vi "6300 laser sweep and oscilloscope.vi"() -> ()   [LabVIEW 2011]
uses:
  <vilib>/Instr/_visa.llb/VISA Open Access Mode.ctl
panel:
  in  "Oscilloscope wait time (ms)":u32
  in  "laser wait time (ms)":u32=1100
  in  "Oscilloscope read time (ms)":u32=4000
  out "error out 2":errorcluster
  in  "Oscilloscope VISA GPIB Resource":refnum<visa-resource-name>="GPIB0::7::INSTR"
  out "error out":errorcluster
  out "WavelengthMin":dbl=1519.01 format="%.2f"
  out "WavelengthMax":dbl=1570.29 format="%.2f"
  out "MaxSlewRate":dbl=23.9 format="%.2f"
  in  "StartSweep":bool
  in  "ReturnSlewrate":dbl=23.9 format="%.2f"
  in  "ForwardSlewrate":dbl=23.9 format="%.2f"
  in  "StopWavelength":dbl=1570.29 format="%.2f"
  in  "StartWavelength":dbl=1519.01 format="%.2f"
  in  "resource name (\"\")":string="GPIB0::10::INSTR"
  # "Sweep Example\n\nStart program with above arrow.\nSet parameters and press StartSweep.\nLaser will reset to the start wavelength then sweep to the stop wavelength."
  # "Min"
  # "Max"
  # "Max"
  # "Set up for GPIB address 1.  Change as needed."
  # "Reference Value:\nFor 2.2s, 4Msa/s:\nlaser wait time: 1100ms;\noscilloscope read time: 4000ms;\n\nFor 2s, 400Ksa/s;\nlaser wait time: 1000ms \noscilloscope read time: \n\nFor 5s, 5Mpts oscilloscope setting:\nlaser wait time: 2600ms;\nOscilloscope read time: 8000ms;\n\nFor 20s, 10Mpts setting:\nlaser wait time: 10500ms;\nOscilloscope read time: 35000ms;\nf\nFor 50s, 200Ksa/s setting:\nlaser wait time: 25000ms\nOscilloscope read time: 85000ms;\nChannel offset:\nCH1:\nCH2:\nCH3:\nCH4:"
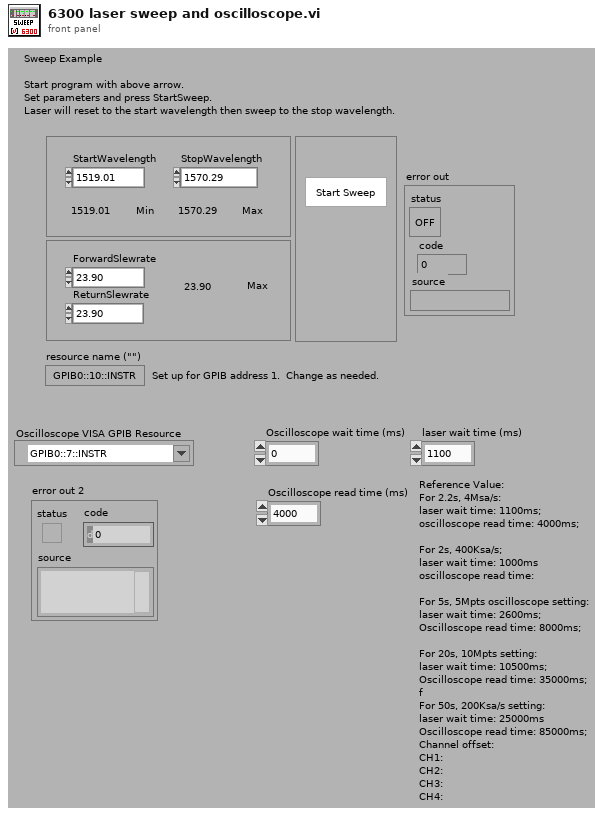
[diagram p1: front panel]
types:
  T1 = enum16{"Diode Current", "Diode Temperature", "Piezo Volt", "Wavelength", "Forward Slew Rate", "Return Slew Rate", "Scan Start Wavelength", "Scan Stop Wavelength", "MaxSlewRate", "Wavelength Max", "Wavelength Min"}
  T2 = enum16{"Diode Current", "Diode Temperature", "Piezo Volt", "Wavelength", "Forward Slewrate", "Return Slewrate", "Scan Start Wavelength", "Scan Stop Wavelength", "Wavelength Max", "Wavelength Min", "Constant Power On", "Constant Power Off"}
  T3 = enum16{"Scan Reset", "Scan Start", "Scan Stop", "Laser On", "Laser Off", "Laser State?", "Track Off"}
  T4 = enum16{"Identification Query", "Operation Complete Query"}
  T5 = typedef "VISA Open Access Mode.ctl" = u32
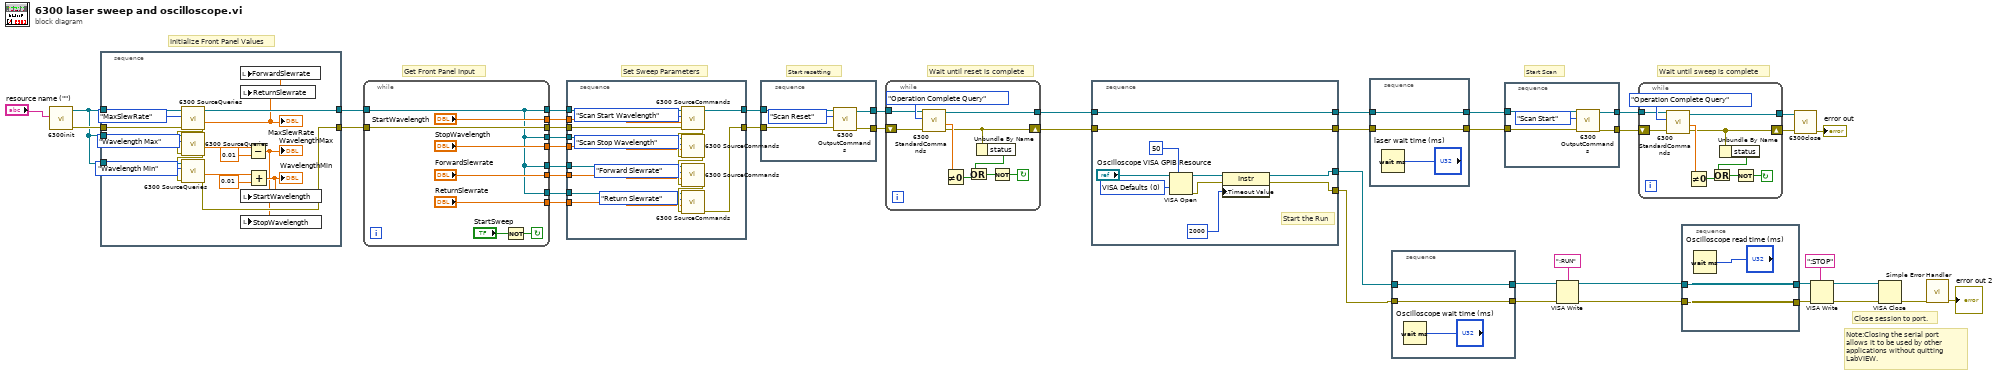
[diagram p0: block diagram]
diagram:
  # "Note:Closing the serial port allows it to be used by other applications without quitting LabVIEW."
  # "Close session to port."
  # "Initialize Front Panel Values"
  # "Wait until sweep is complete"
  # "Start Scan"
  # "Wait until reset is complete"
  # "Start resetting"
  # "Set Sweep Parameters"
  # "Get Front Panel Input"
  n1 = call <instrlib>:"6300init.vi"("resource name (\"\")"="resource name (\"\")") -> ("error out"=w25:errorcluster, "dup VISA session"=w22:refnum<visa-resource-name>)  [unwired: 9 in]
  n2 = stacked-sequence {
    tunnel: w22 -> [w57]
    tunnel: w25 -> [w56]
    tunnel: [w57] -> w24
    tunnel: [w51] -> w23
    tunnel: w22 -> [w55]
    tunnel: w22 -> [w54]
    frame #0 {
      n3 = call <instrlib>:"6300 SourceQueries.VI"("error in"=w56, "Setpoint to Query?"=T1."MaxSlewRate", "VISA session"=w57) -> ("error out"=w53:errorcluster, "Returned Number"=w44:dbl)  [unwired: 5 in, 2 out]
      "MaxSlewRate" <- w44
      n4 = call <instrlib>:"6300 SourceQueries.VI"("error in"=w53, "Setpoint to Query?"=T1."Wavelength Max", "VISA session"=w55) -> ("error out"=w52:errorcluster, "Returned Number"=w47:dbl)  [unwired: 5 in, 2 out]
      n5 = call <instrlib>:"6300 SourceQueries.VI"("error in"=w52, "Setpoint to Query?"=T1."Wavelength Min", "VISA session"=w54) -> ("error out"=w51:errorcluster, "Returned Number"=w48:dbl)  [unwired: 5 in, 2 out]
      n6 = local write "ForwardSlewrate"(w44) -> ()
      n7 = local write "ReturnSlewrate"(w44) -> ()
      n8 = Subtract(x=w47, y=0.01) -> (x-y=w45:dbl)
      "WavelengthMax" <- w45
      n9 = local write "StopWavelength"(w45) -> ()
      n10 = Add(x=w48, y=0.01) -> (x+y=w46:dbl)
      "WavelengthMin" <- w46
      n11 = local write "StartWavelength"(w46) -> ()
    }
  }
  n12 = while {
    tunnel: [w61] -> w34
    tunnel: [w61] -> w35
    tunnel: [w61] -> w36
    tunnel: [w61] -> w37
    tunnel: ["ReturnSlewrate"] -> w39
    tunnel: ["ForwardSlewrate"] -> w40
    tunnel: ["StopWavelength"] -> w41
    tunnel: ["StartWavelength"] -> w42
    tunnel: [w68] -> w38
    tunnel: w23 -> [w68]
    tunnel: w24 -> [w61]
    stop <- w62 continue-if-true
    n13 = Not(x="StartSweep") -> (.not. x?=w62:bool)
  }
  n14 = stacked-sequence {
    tunnel: w42 -> [w83]
    tunnel: w41 -> [w82]
    tunnel: w40 -> [w81]
    tunnel: w39 -> [w80]
    tunnel: w38 -> [w79]
    tunnel: [w78] -> w32
    tunnel: w37 -> [w77]
    tunnel: w36 -> [w76]
    tunnel: w35 -> [w75]
    tunnel: w34 -> [w74]
    tunnel: [w73] -> w33
    frame #0 {
      n15 = call <instrlib>:"6300 SourceCommands.VI"("error in"=w79, "Num Com Parameter"=w83, "Source Command?"=T2."Scan Start Wavelength", "VISA session"=w77) -> ("error out"=w86:errorcluster, "dup VISA session"=w73:refnum<visa-resource-name>)  [unwired: 4 in, 2 out]
      n16 = call <instrlib>:"6300 SourceCommands.VI"("error in"=w86, "Num Com Parameter"=w82, "Source Command?"=T2."Scan Stop Wavelength", "VISA session"=w76) -> ("error out"=w85:errorcluster)  [unwired: 4 in, 3 out]
      n17 = call <instrlib>:"6300 SourceCommands.VI"("error in"=w85, "Num Com Parameter"=w81, "Source Command?"=T2."Forward Slewrate", "VISA session"=w75) -> ("error out"=w84:errorcluster)  [unwired: 4 in, 3 out]
      n18 = call <instrlib>:"6300 SourceCommands.VI"("error in"=w84, "Num Com Parameter"=w80, "Source Command?"=T2."Return Slewrate", "VISA session"=w74) -> ("error out"=w78:errorcluster)  [unwired: 4 in, 3 out]
    }
  }
  n19 = stacked-sequence {
    tunnel: w33 -> [w91]
    tunnel: w32 -> [w90]
    tunnel: [w88] -> w31
    tunnel: [w87] -> w30
    frame #0 {
      n20 = call <instrlib>:"6300 OutputCommands.VI"("error in"=w90, "Output Command?"=T3."Scan Reset", "VISA session"=w91) -> ("error out"=w88:errorcluster, "dup VISA session"=w87:refnum<visa-resource-name>)  [unwired: 3 in, 4 out]
    }
  }
  n21 = while {
    tunnel: [w94] -> w13
    tunnel: w30 -> [w98]
    shift-left: w31 -> [w97]
    shift-right: [w93] -> w12
    stop <- w96 continue-if-true
    n22 = call <instrlib>:"6300 StandardCommands.VI"("error in"=w97, "System Command?"=T4."Operation Complete Query", "VISA session"=w98) -> ("error out"=w93:errorcluster, "Returned Number"=w99:dbl, "dup VISA session"=w94:refnum<visa-resource-name>)  [unwired: 5 in, 1 out]
    n23 = Not Equal To 0?(x=w99) -> (x != 0?=w100:bool)
    n24 = Unbundle By Name(w93) -> ("status"=w92:bool)
    n25 = Or(x=w92, y=w100) -> (x .or. y?=w95:bool)
    n26 = Not(x=w95) -> (.not. x?=w96:bool)
  }
  n27 = stacked-sequence {
    tunnel: w13 -> [w111]
    tunnel: [w111] -> w11
    tunnel: w12 -> [w110]
    tunnel: [w110] -> w9
    tunnel: [w103] -> w7
    tunnel: [w102] -> w6
    frame #0 {
      w109 = T5 0 items=["VISA Defaults"=0, "Exclusive Lock"=1, "Load Configured Settings"=4] ("Access Mode")
      # "Start the Run"
      n28 = VISA Open(timeout (0)=u32 50 ("VISA Open timeout (0)"), access mode=w109, VISA resource name="Oscilloscope VISA GPIB Resource") -> (VISA resource name=w106:refnum<visa-resource-name>, error out=w107:errorcluster)  [unwired: 2 in]
      n29 = property class="Instr"(reference=w106, error in=w107, "General Settings:Timeout Value"=u32 2000) -> (reference out=w103:refnum<visa-resource-name>, error out=w102:errorcluster)
    }
  }
  n30 = stacked-sequence {
    tunnel: w11 -> [w113]
    tunnel: [w113] -> w10
    tunnel: w9 -> [w112]
    tunnel: [w112] -> w8
    frame #0 {
      n31 = Wait (ms)(milliseconds to wait="laser wait time (ms)") -> ()  [unwired: 1 out]
    }
  }
  n32 = stacked-sequence {
    tunnel: w7 -> [w116]
    tunnel: [w116] -> w3
    tunnel: w6 -> [w115]
    tunnel: [w115] -> w4
    frame #0 {
      n33 = Wait (ms)(milliseconds to wait="Oscilloscope wait time (ms)") -> ()  [unwired: 1 out]
    }
  }
  n34 = stacked-sequence {
    tunnel: w10 -> [w122]
    tunnel: w8 -> [w121]
    tunnel: [w119] -> w28
    tunnel: [w118] -> w29
    frame #0 {
      n35 = call <instrlib>:"6300 OutputCommands.VI"("error in"=w121, "Output Command?"=T3."Scan Start", "VISA session"=w122) -> ("error out"=w119:errorcluster, "dup VISA session"=w118:refnum<visa-resource-name>)  [unwired: 3 in, 4 out]
    }
  }
  n36 = VISA Write(VISA resource name=w3, write buffer=":RUN" ("string to write"), error in (no error)=w4) -> (VISA resource name out=w2:refnum<visa-resource-name>, error out=w1:errorcluster)  [unwired: 1 out]
  n37 = while {
    tunnel: [w125] -> w27
    tunnel: w29 -> [w129]
    shift-left: w28 -> [w128]
    shift-right: [w124] -> w26
    stop <- w127 continue-if-true
    n38 = call <instrlib>:"6300 StandardCommands.VI"("error in"=w128, "System Command?"=T4."Operation Complete Query", "VISA session"=w129) -> ("error out"=w124:errorcluster, "Returned Number"=w130:dbl, "dup VISA session"=w125:refnum<visa-resource-name>)  [unwired: 5 in, 1 out]
    n39 = Not Equal To 0?(x=w130) -> (x != 0?=w131:bool)
    n40 = Unbundle By Name(w124) -> ("status"=w123:bool)
    n41 = Or(x=w123, y=w131) -> (x .or. y?=w126:bool)
    n42 = Not(x=w126) -> (.not. x?=w127:bool)
  }
  n43 = stacked-sequence {
    tunnel: w2 -> [w134]
    tunnel: [w134] -> w15
    tunnel: w1 -> [w133]
    tunnel: [w133] -> w14
    frame #0 {
      n44 = Wait (ms)(milliseconds to wait="Oscilloscope read time (ms)") -> ()  [unwired: 1 out]
    }
  }
  n45 = call <instrlib>:"6300close.vi"("error in"=w26, "VISA session"=w27) -> ("error out"=→"error out":errorcluster)  [unwired: 9 in]
  n46 = VISA Write(VISA resource name=w15, write buffer=":STOP" ("string to write"), error in (no error)=w14) -> (VISA resource name out=w16:refnum<visa-resource-name>, error out=w17:errorcluster)  [unwired: 1 out]
  n47 = VISA Close(VISA resource name=w16, error in (no error)=w17) -> (error out=w20:errorcluster)
  n48 = call <vilib>:"Simple Error Handler.vi"("error in (no error)"=w20) -> ("error out"=→"error out 2":errorcluster)  [unwired: 1 in, 7 out]
